vi "SynapseAPI-Set Parameter Value (1D).vi"(0 "URL":string="http://localhost:24414", 5 "Gizmo":string, 7 "Parameter":string, 9 "Values":dbl[](array[numeric]), 11 "error in (no error)":errorcluster) -> (15 "error out":errorcluster)   [LabVIEW 2020]
uses:
  <vilib>/httpClient/PUTBuffer.vi
  <vilib>/httpClient/LabVIEWHTTPClient.lvlib
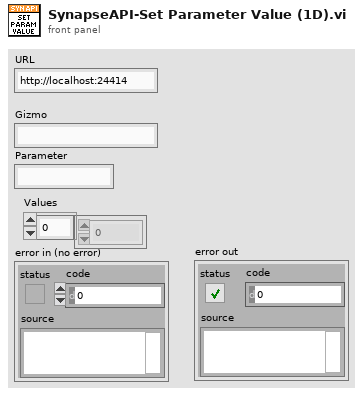
[diagram p1: front panel]
types:
  T1 = typedef "LabVIEWHTTPClient.lvlib/ClientHandle.ctl" = refnum<k1>
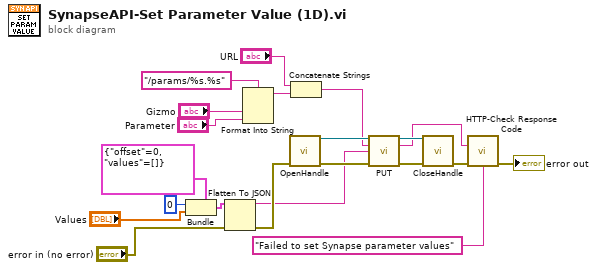
[diagram p0: block diagram]
diagram:
  n1 = Bundle(cluster=cluster{"offset":i32, "values":dbl[]} {"offset"=0, "values"=[]} ("Cluster"), "offset"=0 ("iOffset"), "values"="Values") -> (w10:cluster{"offset":i32, "values":dbl[]})
  n2 = Flatten To JSON(anything=w10, error in (no error)="error in (no error)") -> (JSON string=w7:string, 11:w8:errorcluster)  [unwired: 1 in]
  n3 = Format Into String(format string="/params/%s.%s", "Gizmo", "Parameter") -> (resulting string=w15:string)  [unwired: 2 in, 1 out]
  n4 = call <vilib>:"OpenHandle.vi"("error in (no error)"=w8) -> ("client handle out"=w19:T1, "error out"=w18:errorcluster)  [unwired: 13 in]
  n5 = Concatenate Strings("URL", w15) -> (w17:string)
  n6 = call-poly <vilib>:"PUT.vi"("client handle"=w19, "url"=w17, "buffer"=w7, "error in (no error)"=w18) -> ("client handle out"=w20:T1, "headers"=w3:string, "error out"=w21:errorcluster)  [unwired: 8 in, 1 out]
  n7 = call <vilib>:"CloseHandle.vi"("client handle"=w20, "error in (no error)"=w21) -> ("error out"=w5:errorcluster)  [unwired: 13 in]
  n8 = call "HTTP-Check Response Code.vi"("headers"=w3, "error in"=w5, "message"="Failed to set Synapse parameter values") -> ("error out"=→"error out":errorcluster)  [unwired: 12 in]
